vi "ShooterTest.vi"() -> ()   [LabVIEW 2013]
uses:
  <vilib>/Rock Robotics/SystemInterfaces/Typedef/FPGA_TypedefSolenoidModule.ctl
  <vilib>/Rock Robotics/WPI/Solenoid/WPI_SolenoidChannel.ctl
  <vilib>/Rock Robotics/WPI/Joystick/WPI_JoystickDeviceEnum.ctl
  <vilib>/Rock Robotics/SystemInterfaces/DIO/FPGA_DIOChannel.ctl
  <vilib>/Rock Robotics/SystemInterfaces/Typedef/FPGA_TypedefDigitalModule.ctl
  <vilib>/Rock Robotics/SystemInterfaces/DIO/FPGA_DIORelayChannel.ctl
  Robot_Framework_2014/SingleSolenoidAction.ctl
  <vilib>/Rock Robotics/WPI/Solenoid/WPI_SolenoidOpenSingle.vi
panel:
  in  "Firing Channel 2":T1=enum."Solenoid 7"
  in  "Firing Module 2":T2
  in  "Kicker Module":T2
  in  "Kicker Channel":T1
  in  "Firing Channel":T1=enum."Solenoid 3"
  in  "Firing Module":T2
  # "BUTTON 5\nL1"
  # "BUTTON 6\nR1"
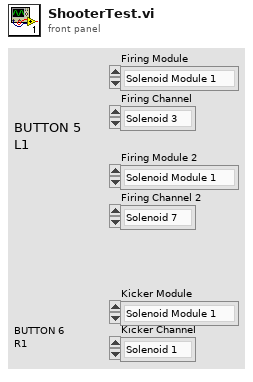
[diagram p1: front panel]
types:
  T1 = typedef "WPI_SolenoidChannel.ctl" = enum8{"Solenoid 1", "Solenoid 2", "Solenoid 3", "Solenoid 4", "Solenoid 5", "Solenoid 6", "Solenoid 7", "Solenoid 8", "Invalid"}
  T2 = typedef "FPGA_TypedefSolenoidModule.ctl" = enum16{"Solenoid Module 1", "Solenoid Module 2"}
  T3 = typedef "SingleSolenoidAction.ctl" = enum16{"Init", "SetState", "Disable"}
  T4 = typedef "FPGA_DIORelayChannel.ctl" = enum8{"Relay 1", "Relay 2", "Relay 3", "Relay 4", "Relay 5", "Relay 6", "Relay 7", "Relay 8", "Invalid"}
  T5 = typedef "FPGA_TypedefDigitalModule.ctl" = enum16{"Digital Module 1", "Digital Module 2"}
  T6 = typedef "FPGA_DIOChannel.ctl" = enum8{"DIO 1", "DIO 2", "DIO 3", "DIO 4", "DIO 5", "DIO 6", "DIO 7", "DIO 8", "DIO 9", "DIO 10", "DIO 11", "DIO 12", "DIO 13", "DIO 14", "Invalid"}
  T7 = typedef "WPI_JoystickDeviceEnum.ctl" = enum16{"USB 1", "USB 2", "USB 3", "USB 4", "Kinect 1", "Kinect 2"}
  T8 = typedef "WPI_JoystickDevRef.ctl" = cluster{"Device":T7}
  T9 = typedef "WPI_SolenoidDevRef.ctl" = cluster{"DevStatus":errorcluster, "Solenoid Module":T2, "Forward Solenoid Channel":T1, "Reverse Solenoid Channel":T1}
  T10 = typedef "WPI_CompressorDevRef.ctl" = cluster{"DevStatus":errorcluster, "DigitalInputDevRef":T11, "RelayDevRef":T12}
  T11 = typedef "WPI_DigitalInputDevRef.ctl" = cluster{"DevStatus":errorcluster, "DIO Channel":T6, "Digital Module":T5}
  T12 = typedef "WPI_RelayDevRef.ctl" = cluster{"DevStatus":errorcluster, "Relay Channel":T4, "Digital Module":T5, "Relay Direction":T13}
  T13 = typedef "WPI_RelayDirection.ctl" = enum16{"Both directions", "Forward only", "Reverse only"}
  T14 = typedef "WPI_JoystickButtonState.ctl" = cluster{"Button 1":bool, "Button 2":bool, "Button 3":bool, "Button 4":bool, "Button 5":bool, "Button 6":bool, "Button 7":bool, "Button 8":bool, "Button 9":bool, "Button 10":bool, "Button 11":bool, "Button 12":bool}
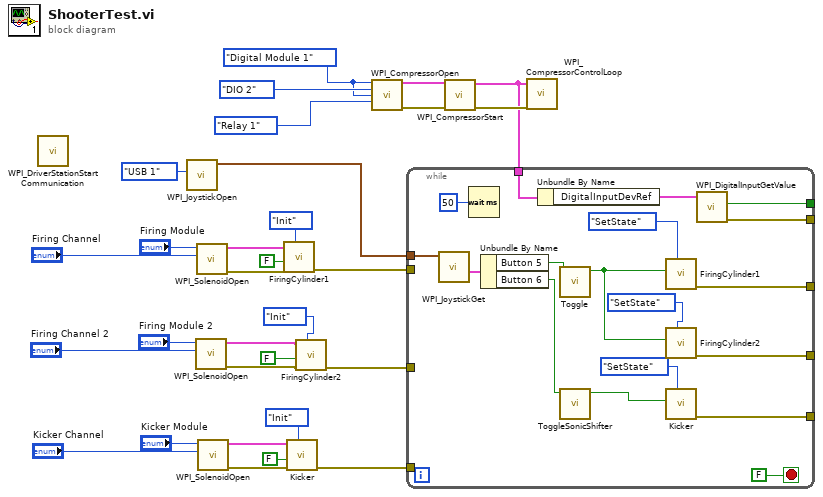
[diagram p0: block diagram]
diagram:
  w13 = FPGA_TypedefDigitalModule."Digital Module 1" ("Pressure Switch Digital Module (Module 1)")
  n1 = call <vilib>:"WPI_DriverStationStart Communication.vi"() -> ()  [unwired: 12 in]
  n2 = call <vilib>:"WPI_JoystickOpen.vi"("JoystickDevice"=WPI_JoystickDeviceEnum."USB 1") -> ("JoystickDevRef"=w16:T8)  [unwired: 10 in]
  n3 = call-poly <vilib>:"WPI_SolenoidOpen.vi"("Solenoid Channel"="Firing Channel 2", "Solenoid Module (Module 1)"="Firing Module 2") -> ("error out"=w4:errorcluster, "SolenoidDevRef"=w5:T9)  [unwired: 8 in]
  n4 = call-poly <vilib>:"WPI_SolenoidOpen.vi"("Solenoid Channel"="Firing Channel", "Solenoid Module (Module 1)"="Firing Module") -> ("error out"=w18:errorcluster, "SolenoidDevRef"=w19:T9)  [unwired: 8 in]
  n5 = call-poly <vilib>:"WPI_SolenoidOpen.vi"("Solenoid Channel"="Kicker Channel", "Solenoid Module (Module 1)"="Kicker Module") -> ("error out"=w17:errorcluster, "SolenoidDevRef"=w20:T9)  [unwired: 8 in]
  n6 = call "FiringCylinder1.vi"("Action"=SingleSolenoidAction."Init", "error in (no error)"=w18, "Default Position"=FALSE, "SolenoidDevRef"=w19) -> ("error out"=w28:errorcluster)  [unwired: 7 in]
  n7 = call "Kicker.vi"("Action"=SingleSolenoidAction."Init", "error in (no error)"=w17, "Default Position"=FALSE, "SolenoidDevRef"=w20) -> ("error out"=w27:errorcluster)  [unwired: 7 in]
  n8 = call "FiringCylinder2.vi"("Action"=SingleSolenoidAction."Init", "error in (no error)"=w4, "Default Position"=FALSE, "SolenoidDevRef"=w5) -> ("error out"=w3:errorcluster)  [unwired: 7 in]
  n9 = call <vilib>:"WPI_CompressorOpen.vi"("Pressure Switch Digital Module (Module 1)"=w13, "Pressure Switch DIO Channel"=FPGA_DIOChannel."DIO 2", "Relay Digital Module (Module 1)"=w13, "Relay Channel"=FPGA_DIORelayChannel."Relay 1") -> ("CompressorDevRef"=w11:T10, "error out"=w10:errorcluster)  [unwired: 10 in]
  n10 = call <vilib>:"WPI_CompressorStart.vi"("error in (no error)"=w10, "CompressorDevRef"=w11) -> ("error out"=w9:errorcluster, "CompressorDevRef"=w1:T10)  [unwired: 8 in]
  n11 = while {
    tunnel: w28 -> [_]
    tunnel: w27 -> [_]
    tunnel: w16 -> [w45]
    tunnel: w3 -> [_]
    tunnel: [w37] -> _
    tunnel: [w36] -> _
    tunnel: [w35] -> _
    tunnel: w1 -> [w34]
    tunnel: [w32] -> _
    tunnel: [w31] -> _
    stop <- FALSE stop-if-true
    n12 = call <vilib>:"WPI_JoystickGet.vi"("JoystickDevRef"=w45) -> ("Buttons"=w44:T14)  [unwired: 4 in, 2 out]
    n13 = Wait (ms)(milliseconds to wait=u32 50) -> ()  [unwired: 1 out]
    n14 = Unbundle By Name(w44) -> ("Button 5"=w43:bool, "Button 6"=w42:bool)
    n15 = Unbundle By Name(w34) -> ("DigitalInputDevRef"=w33:T11)
    n16 = call "Toggle.vi"("RawInput"=w43) -> ("ToggleState"=w39:bool)  [unwired: 9 in, 1 out]
    n17 = call "ToggleSonicShifter.vi"("cSonicShifter"=w42) -> ("Actuate?"=w41:bool)  [unwired: 9 in, 1 out]
    n18 = call "FiringCylinder1.vi"("Action"=SingleSolenoidAction."SetState", "Actuate?"=w39) -> ("error out"=w37:errorcluster)  [unwired: 9 in]
    n19 = call "FiringCylinder2.vi"("Action"=SingleSolenoidAction."SetState", "Actuate?"=w39) -> ("error out"=w36:errorcluster)  [unwired: 9 in]
    n20 = call "Kicker.vi"("Action"=SingleSolenoidAction."SetState", "Actuate?"=w41) -> ("error out"=w35:errorcluster)  [unwired: 9 in]
    n21 = call <vilib>:"WPI_DigitalInputGetValue.vi"("DigitalInputDevRef"=w33) -> ("error out"=w31:errorcluster, "Value"=w32:bool)  [unwired: 8 in, 1 out]
  }
  n22 = call <vilib>:"WPI_CompressorControlLoop.vi"("error in (no error)"=w9, "CompressorDevRef"=w1) -> ()  [unwired: 10 in]
